vi "delta deg.vi"(1 "array phase":dbl[](array[numeric])) -> (0 "delta phase":dbl[](array[numeric]))   [LabVIEW 2021]
uses:
  <vilib>/Analysis/coordinate.llb/Angle Units.ctl
  <vilib>/Analysis/coordinate.llb/Angle Range (Degree).ctl
  <vilib>/Analysis/coordinate.llb/Wrap Angle (array).vi
  <vilib>/Analysis/NI_AAL_Angle.lvlib
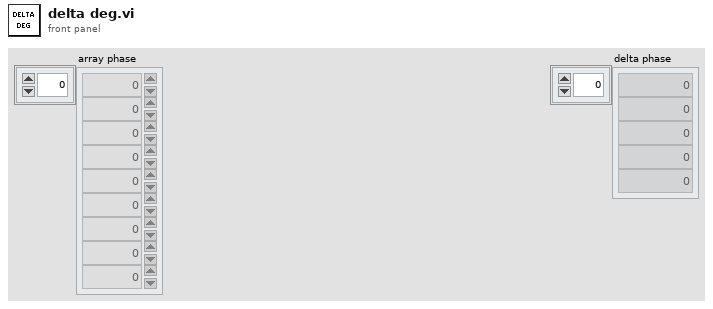
[diagram p1: front panel]
types:
  T1 = typedef "NI_AAL_Angle.lvlib/Angle Range (Degree).ctl" = u16
  T2 = typedef "NI_AAL_Angle.lvlib/Angle Units.ctl" = i32
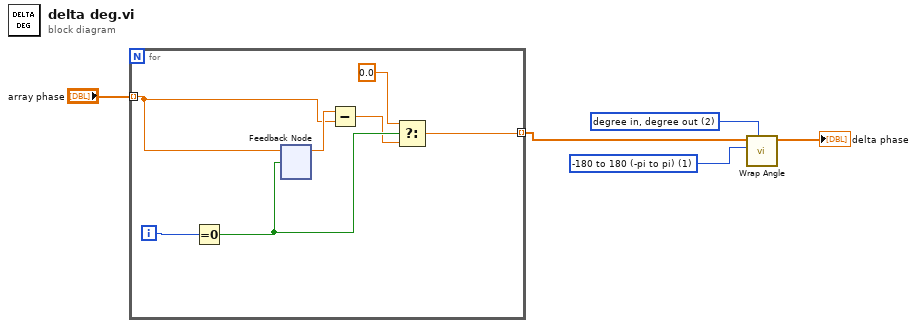
[diagram p0: block diagram]
diagram:
  w1 = T1 1 items=["none", "-180 to 180 (-pi to pi)", "0 to 360 (0 to 2pi)"] ("angle range")
  w2 = T2 2 items=["radian in, radian out", "radian in, degree out", "degree in, degree out", "degree in, radian out"] ("angle units")
  n1 = for {
    tunnel: "array phase" -> [w8] mode=indexing
    tunnel: [w6] -> w4 mode=indexing
    i -> [w12]
    n2 = Equal To 0?(x=w12) -> (x = 0?=w11:bool)
    n3 = feedback-in #1(w8, w11) -> ()
    n4 = feedback #1() -> (w9:dbl)  [unwired: 1 in]
    n5 = Subtract(x=w9, y=w8) -> (x-y=w7:dbl)
    n6 = Select(t=0.0, s=w11, f=w7) -> (s? t:f=w6:dbl)
  }
  n7 = call-poly <vilib>:"Wrap Angle.vi"("angle units"=w2, "angle range"=w1, "Angle In"=w4) -> ("Angle Out"=→"delta phase":dbl[])  [unwired: 7 in, 1 out]
